vi "Write Digital Port.vi"(8 "error in (no error)":errorcluster, 10 "Relay Mode":bool[](array[boolean]), 11 "Sim DIO in":refnum<class "Sim DIO.lvclass">) -> (0 "error out":errorcluster, 3 "Sim DIO out":refnum<class "Sim DIO.lvclass">)   [LabVIEW 2019, in "Concrete.lvlib" / "Sim DIO.lvclass"]
uses:
  Sim DIO.lvclass
  Harware Abstraction/DIO/DIO.lvclass
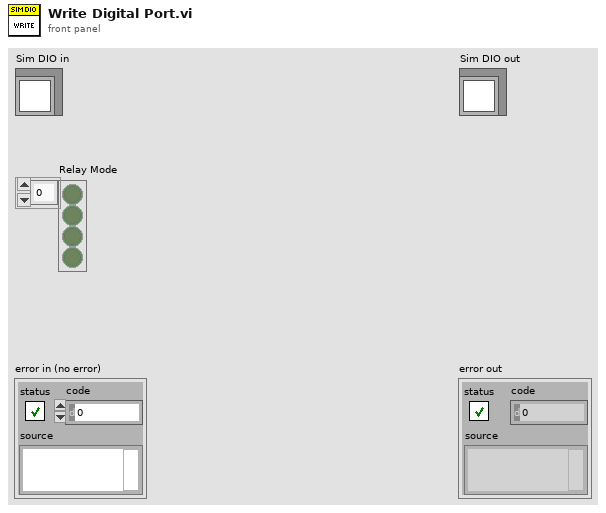
[diagram p1: front panel]
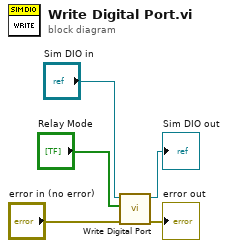
[diagram p0: block diagram]
diagram:
  n1 = call-parent "Write Digital Port.vi"("error in (no error)"="error in (no error)", "Relay Mode"="Relay Mode", "DIO in"="Sim DIO in") -> ("error out"=→"error out":errorcluster, "DIO out"=→"Sim DIO out":refnum<class "Sim DIO.lvclass">)  [unwired: 7 in]
